vi "TrapTcpError.vi"(7 "Controller":refnum<data-value>, 8 "error in (no error)":errorcluster, 9 "connected":refnum<data-value>, 10 "Qbus in":refnum<data-value>, 11 "MainLoopQ":refnum<data-value>) -> (0 "error out":errorcluster)   [LabVIEW 2017]
uses:
  <vilib>/addons/InsightCM/Utilities/Qbus/Qbus/controls/Qbus_Qdata.ctl
  <vilib>/addons/InsightCM/Utilities/Qbus/Qbus/controls/Qbus_QbusData.ctl
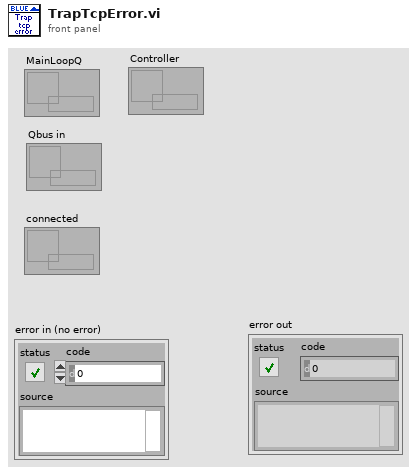
[diagram p1: front panel]
types:
  T1 = typedef "DvrRefrence.ctl" = refnum<data-value>
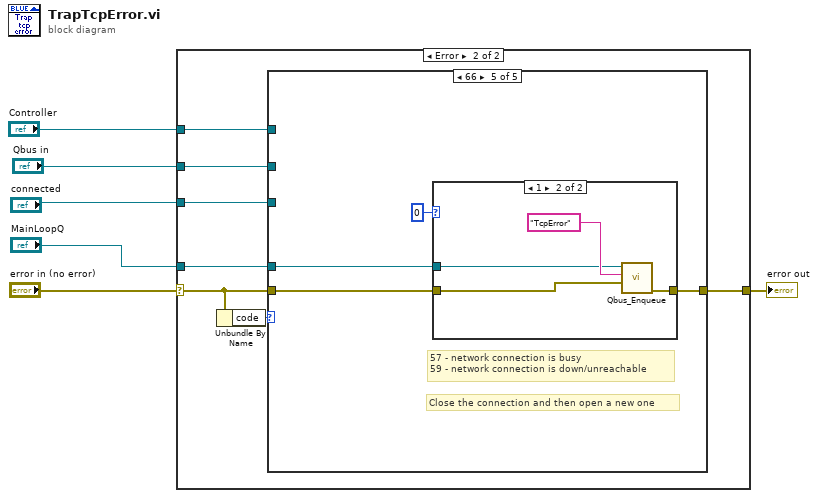
[diagram p0: block diagram]
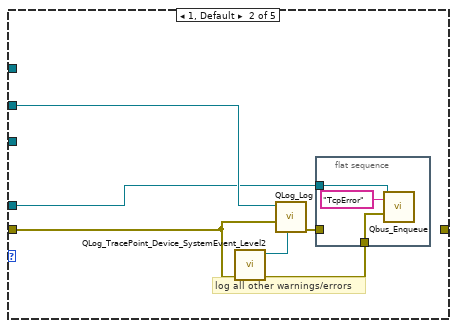
[diagram p4: hidden frame]
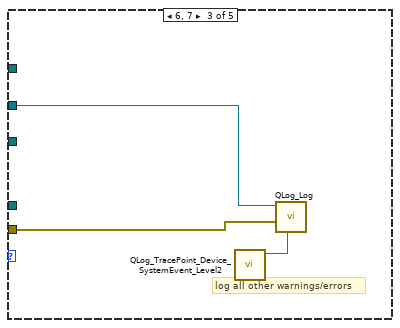
[diagram p5: hidden frame]
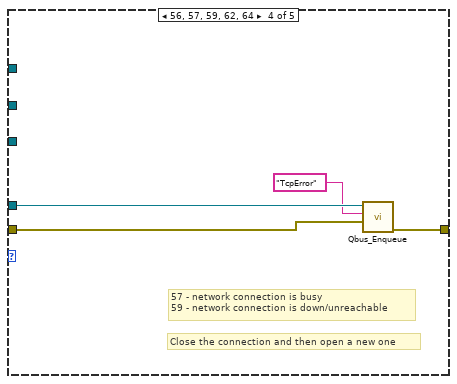
[diagram p6: hidden frame]
diagram:
  n1 = case shown="Error" "error in (no error)" {
    selector: "error in (no error)" -> [w7 w13]
    tunnel: "MainLoopQ" -> [_ w12]
    tunnel: [w7 w11] -> w5
    tunnel: "connected" -> [_ w10]
    tunnel: "Qbus in" -> [_ w9]
    tunnel: "Controller" -> [_ w8]
    frame No Error {
    }
    frame Error {
      n2 = Unbundle By Name(w13) -> ("code"=w14:i32)
      n3 = case shown="66" w14 {
        tunnel: w13 -> [w15 w18 w24 w30 w34]
        tunnel: w12 -> [_ w16 _ w29 w33]
        tunnel: [w15 _ _ w28 w32] -> w11
        tunnel: w10 -> [_ _ _ _ _]
        tunnel: w9 -> [_ w19 w25 _ _]
        tunnel: w8 -> [_ _ _ _ _]
        frame 0 {
        }
        frame 1, Default {
          # "log all other warnings/errors"
          n4 = call <vilib>:"QLog_TracePoint_Device_SystemEvent_Level2.vi"() -> ("DvrRef"=w20:T1)  [unwired: 11 in]
          n5 = call <vilib>:"QLog_Log.vi"("DvrRef"=w20, "Value"=w18, "Qbus in"=w19) -> ("error out"=w17:errorcluster)  [unwired: 7 in, 1 out]
          n6 = flat-sequence {
            tunnel: w18 -> [w21]
            tunnel: w17 -> [_]
            tunnel: w16 -> [w23]
            frame #0 {
              n7 = call <vilib>:"Qbus_Enqueue.vi"("MsgValue"=w21, "MsgName"="TcpError", "Q in"=w23) -> ()  [unwired: 7 in, 2 out]
            }
          }
        }
        frame 6, 7 {
          # "log all other warnings/errors"
          n8 = call <vilib>:"QLog_TracePoint_Device_SystemEvent_Level2.vi"() -> ("DvrRef"=w26:T1)  [unwired: 11 in]
          n9 = call <vilib>:"QLog_Log.vi"("DvrRef"=w26, "Value"=w24, "Qbus in"=w25) -> ()  [unwired: 7 in, 2 out]
        }
        frame 56, 57, 59, 62, 64 {
          # "Close the connection and then open a new one"
          # "57 - network connection is busy\n59 - network connection is down/unreachable"
          n10 = call <vilib>:"Qbus_Enqueue.vi"("MsgValue"=w30, "MsgName"="TcpError", "Q in"=w29) -> ("error out"=w28:errorcluster)  [unwired: 7 in, 1 out]
        }
        frame 66 {
          # "Close the connection and then open a new one"
          # "57 - network connection is busy\n59 - network connection is down/unreachable"
          n11 = case shown="1" 0 {
            tunnel: w34 -> [_ w37]
            tunnel: w33 -> [_ w36]
            tunnel: [_ w35] -> w32
            frame 0, Default {
            }
            frame 1 {
              n12 = call <vilib>:"Qbus_Enqueue.vi"("MsgValue"=w37, "MsgName"="TcpError", "Q in"=w36) -> ("error out"=w35:errorcluster)  [unwired: 7 in, 1 out]
            }
          }
        }
      }
    }
  }
  "error out" <- w5
